vi "Read from Measurement File.vi"() -> ()   [LabVIEW 2023]
panel:
  out "Waveform Graph":dynamicdata(graph)
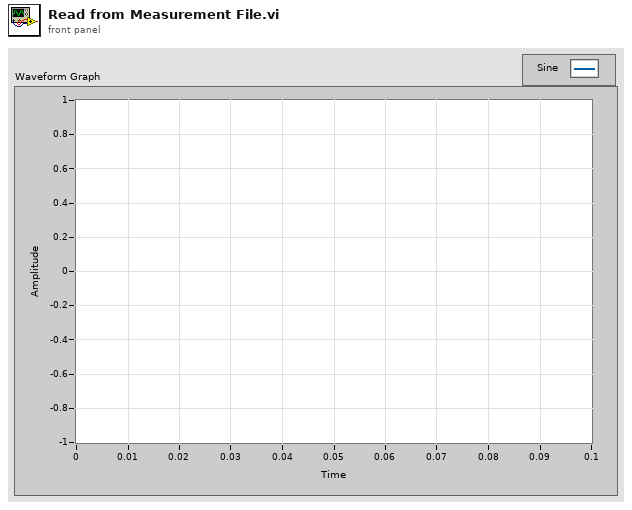
[diagram p1: front panel]
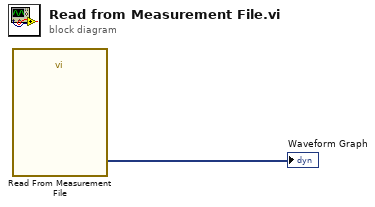
[diagram p0: block diagram]
diagram:
  n1 = call "Read From Measurement File"() -> ("Signals"=→"Waveform Graph":dynamicdata)  [unwired: 6 in, 5 out]
